vi "Get Temperature Status.vi"(7 "CoolerVolts":sgl, 9 "AmbientTemp":sgl, 10 "TargetTemp":sgl, 11 "SensorTemp":sgl) -> (1 "AmbientTemp out":sgl, 2 "TargetTemp out":sgl, 3 "SensorTemp out":sgl, 4 "function return":u32, 5 "CoolerVolts out":sgl)   [LabVIEW 2018, in "AndorSDK.lvlib"]
doc: "EXPNETTYPE unsigned int WINAPI GetTemperatureStatus(float * SensorTemp, float * TargetTemp, float * AmbientTemp, float * CoolerVolts);"
uses:
  AndorSDK.lvlib
  ATMCD32D.dll
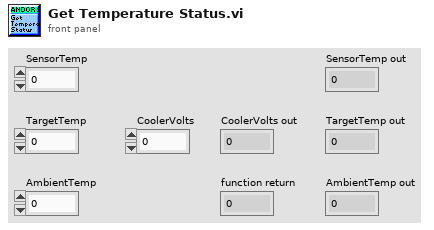
[diagram p1: front panel]
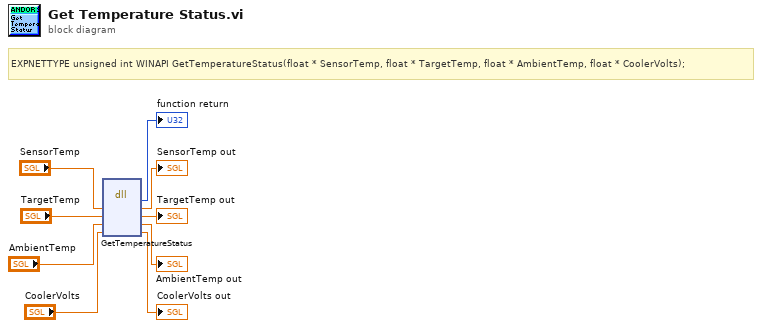
[diagram p0: block diagram]
diagram:
  # "EXPNETTYPE unsigned int WINAPI GetTemperatureStatus(float * SensorTemp, float * TargetTemp, float * AmbientTemp, float * CoolerVolts);"
  n1 = dll-call lib="PTH2babs E\nPersönliches02 - Arbeit03-HiwijobsLabviewCodelibANDOR\tAndor SDK\nATMCD32D.*" fn="GetTemperatureStatus"("SensorTemp"="SensorTemp", "TargetTemp"="TargetTemp", "AmbientTemp"="AmbientTemp", "CoolerVolts"="CoolerVolts") -> (→"function return":u32, "SensorTemp"=→"SensorTemp out":sgl, "TargetTemp"=→"TargetTemp out":sgl, "AmbientTemp"=→"AmbientTemp out":sgl, "CoolerVolts"=→"CoolerVolts out":sgl)  [unwired: 3 in, 2 out]
